vi "TxBfrDat - Init Packet Page.vi"(6 "Tx Buffered Data Packet Refs":T1, 8 "error in (no error)":errorcluster, 11 "Node Ptr In":T2 format="%.0x") -> (0 "error out":errorcluster, 3 "Node Ptr Out":T2 format="%.0x")   [LabVIEW 2016, in "UDP-Custom-Device System Explorer.lvlib"]
uses:
  UDP-Custom-Device System Explorer.lvlib
  <vilib>/NI Veristand/Custom Device API/Custom Device Item Ref.ctl
  Types/Page References/Refs - Tx Buffered Data Packet Page.ctl
  <vilib>/NI VeriStand/Custom Device API/Custom Device API.lvlib
  Property Accessors/Shared Packet Accessors.lvlib
  Property Accessors/Buffered Data Packet.lvlib
  Property Accessors/Tx Packet Accessors.lvlib
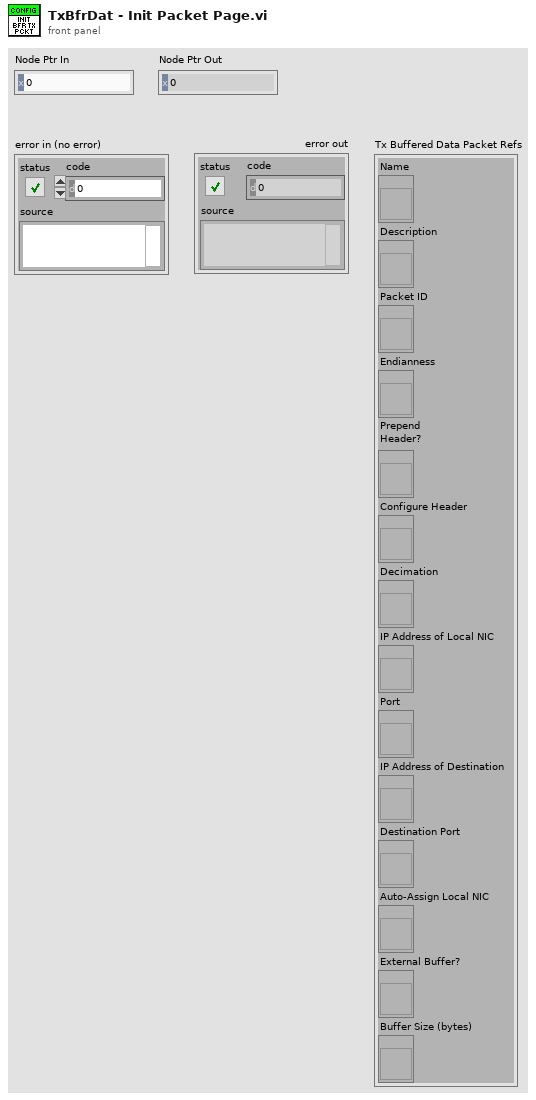
[diagram p1: front panel]
types:
  T1 = typedef "UDP-Custom-Device System Explorer.lvlib/Refs - Tx Buffered Data Packet Page.ctl" = cluster{"Name":refnum<vi>, "Description":refnum<vi>, "Packet ID":refnum<vi>, "Endianness":refnum<vi>, "Prepend\nHeader?":refnum<vi>, "Configure Header":refnum<vi>, "Decimation":refnum<vi>, "IP Address of Local NIC":refnum<vi>, "Port":refnum<vi>, "IP Address of Destination":refnum<vi>, "Destination Port":refnum<vi>, "Auto-Assign Local NIC":refnum<vi>, "External Buffer?":refnum<vi>, "Buffer Size (bytes)":refnum<vi>}
  T2 = typedef "Custom Device API.lvlib/Custom Device Item Ref.ctl" = u64
  T3 = enum8{"Enabled", "Disabled", "Disabled and Grayed Out"}
  T4 = typedef "Custom Device API.lvlib/Custom Device Item Info.ctl" = cluster{"Name":string, "Is Channel":bool, "GUID":string, "Is Waveform":bool}
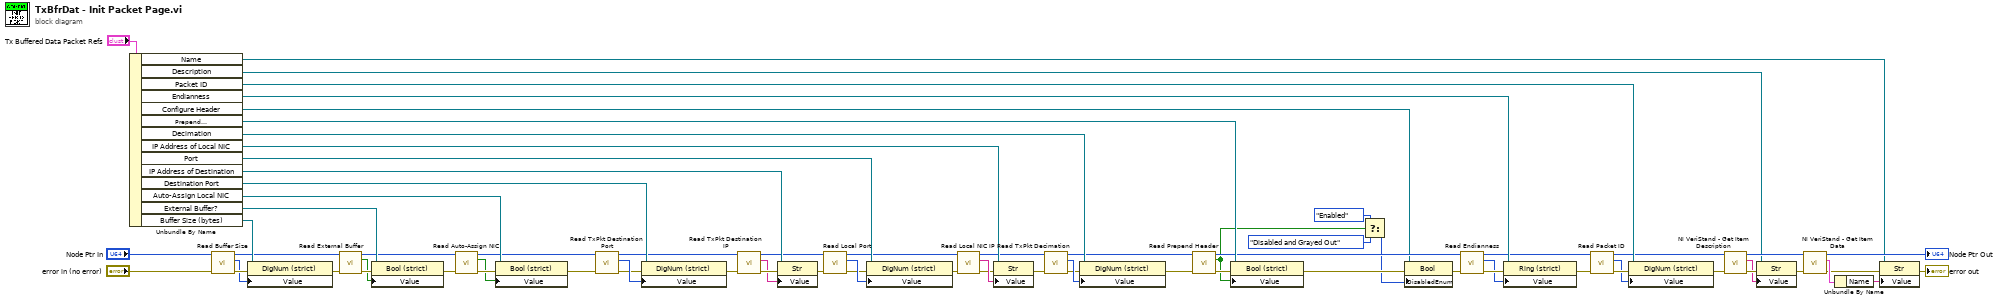
[diagram p0: block diagram]
diagram:
  n1 = Unbundle By Name("Tx Buffered Data Packet Refs") -> ("Name"=w64:refnum<vi>, "Description"=w63:refnum<vi>, "Packet ID"=w62:refnum<vi>, "Endianness"=w55:refnum<vi>, "Configure Header"=w44:refnum<vi>, "Prepend\nHeader?"=w52:refnum<vi>, "Decimation"=w42:refnum<vi>, "IP Address of Local NIC"=w37:refnum<vi>, "Port"=w31:refnum<vi>, "IP Address of Destination"=w24:refnum<vi>, "Destination Port"=w21:refnum<vi>, "Auto-Assign Local NIC"=w16:refnum<vi>, "External Buffer?"=w12:refnum<vi>, "Buffer Size (bytes)"=w10:refnum<vi>)
  n2 = call "Read Buffer Size.vi"("error in (no error)"="error in (no error)", "Node Ptr"="Node Ptr In") -> ("error out"=w2:errorcluster, "Buffer Size"=w1:u32, "Node Ptr out"=w9:T2)  [unwired: 7 in]
  n3 = property class="DigNum (strict)"(reference=w10, error in=w2, "Value"=w1) -> (error out=w7:errorcluster)  [unwired: 1 out]
  n4 = call "Read External Buffer.vi"("error in (no error)"=w7, "Node Ptr"=w9) -> ("error out"=w6:errorcluster, "External Buffer"=w5:bool, "Node Ptr out"=w8:T2)  [unwired: 7 in]
  n5 = property class="Bool (strict)"(reference=w12, error in=w6, "Value"=w5) -> (error out=w11:errorcluster)  [unwired: 1 out]
  n6 = call "Read Auto-Assign NIC.vi"("error in (no error)"=w11, "Node Ptr"=w8) -> ("error out"=w15:errorcluster, "Auto-Assign NIC"=w14:bool, "Node Ptr out"=w13:T2)  [unwired: 7 in]
  n7 = property class="Bool (strict)"(reference=w16, error in=w15, "Value"=w14) -> (error out=w17:errorcluster)  [unwired: 1 out]
  n8 = call "Read TxPkt Destination Port.vi"("error in (no error)"=w17, "Node Ptr"=w13) -> ("error out"=w19:errorcluster, "Destination Port"=w20:u16, "Node Ptr out"=w18:T2)  [unwired: 7 in]
  n9 = property class="DigNum (strict)"(reference=w21, error in=w19, "Value"=w20) -> (error out=w26:errorcluster)  [unwired: 1 out]
  n10 = call "Read TxPkt Destination IP.vi"("error in (no error)"=w26, "Node Ptr"=w18) -> ("error out"=w25:errorcluster, "Destination IP"=w23:string, "Node Ptr out"=w22:T2)  [unwired: 7 in]
  n11 = property class="Str"(reference=w24, error in=w25, "Value"=w23) -> (error out=w27:errorcluster)  [unwired: 1 out]
  n12 = call "Read Local Port.vi"("error in (no error)"=w27, "Node Ptr"=w22) -> ("error out"=w29:errorcluster, "Port"=w30:u16, "Node Ptr out"=w28:T2)  [unwired: 7 in]
  n13 = property class="DigNum (strict)"(reference=w31, error in=w29, "Value"=w30) -> (error out=w32:errorcluster)  [unwired: 1 out]
  n14 = call "Read Local NIC IP.vi"("error in (no error)"=w32, "Node Ptr"=w28) -> ("error out"=w34:errorcluster, "IP Address of Local NIC"=w35:string, "Node Ptr out"=w33:T2)  [unwired: 7 in]
  n15 = property class="Str"(reference=w37, error in=w34, "Value"=w35) -> (error out=w36:errorcluster)  [unwired: 1 out]
  n16 = call "Read TxPkt Decimation.vi"("error in (no error)"=w36, "Node Ptr"=w33) -> ("error out"=w40:errorcluster, "Decimation"=w41:u16, "Node Ptr out"=w38:T2)  [unwired: 7 in]
  n17 = property class="DigNum (strict)"(reference=w42, error in=w40, "Value"=w41) -> (error out=w39:errorcluster)  [unwired: 1 out]
  n18 = call "Read Prepend Header.vi"("error in (no error)"=w39, "Node Ptr"=w38) -> ("error out"=w51:errorcluster, "Prepend Header"=w47:bool, "Node Ptr out"=w50:T2)  [unwired: 7 in]
  n19 = property class="Bool (strict)"(reference=w52, error in=w51, "Value"=w47) -> (error out=w46:errorcluster)  [unwired: 1 out]
  n20 = Select(t=T3."Enabled" ("Disabled"), s=w47, f=T3."Disabled and Grayed Out" ("Disabled")) -> (s? t:f=w43:T3)
  n21 = property class="Bool"(reference=w44, error in=w46, "DisabledEnum"=w43) -> (error out=w45:errorcluster)  [unwired: 1 out]
  n22 = call "Read Endianness.vi"("error in (no error)"=w45, "Node Ptr"=w50) -> ("error out"=w56:errorcluster, "Endianness"=w54:u16, "Node Ptr out"=w53:T2)  [unwired: 7 in]
  n23 = property class="Ring (strict)"(reference=w55, error in=w56, "Value"=w54) -> (error out=w57:errorcluster)  [unwired: 1 out]
  n24 = call "Read Packet ID.vi"("error in (no error)"=w57, "Node Ptr"=w53) -> ("error out"=w59:errorcluster, "Packet ID"=w58:i32, "Node Ptr out"=w60:T2)  [unwired: 7 in]
  n25 = property class="DigNum (strict)"(reference=w62, error in=w59, "Value"=w58) -> (error out=w61:errorcluster)  [unwired: 1 out]
  n26 = call <vilib>:"NI VeriStand - Get Item Description.vi"("error in (no error)"=w61, "Item Ref in"=w60) -> ("error out"=w71:errorcluster, "Description"=w70:string, "Item Ref out"=w68:T2)  [unwired: 7 out]
  n27 = property class="Str"(reference=w63, error in=w71, "Value"=w70) -> (error out=w69:errorcluster)  [unwired: 1 out]
  n28 = call <vilib>:"NI VeriStand - Get Item Data.vi"("error in (no error)"=w69, "Item Ref in"=w68) -> ("error out"=w72:errorcluster, "Item Info"=w73:T4, "Item Ref out"=→"Node Ptr Out":T2)  [unwired: 6 in, 1 out]
  n29 = Unbundle By Name(w73) -> ("Name"=w67:string)
  n30 = property class="Str"(reference=w64, error in=w72, "Value"=w67) -> (error out=→"error out":errorcluster)  [unwired: 1 out]
